vi "Setup.vi"(8 "Error In":errorcluster, 9 "Password":string, 10 "Username":string, 11 "Address":string) -> (0 "Error Out":errorcluster, 3 "Sesssion":refnum<class "Session.lvclass">)   [LabVIEW 2018, in "Tests.lvlib" / "SFTP.lvlib"]
uses:
  SFTP.lvlib
  src/Toolkit/API/Session/Session.lvclass
  src/Toolkit/API/Session/Support/Password Authentication.vi
  src/Toolkit/API/SSH/SSH.lvclass
  Tests.lvlib
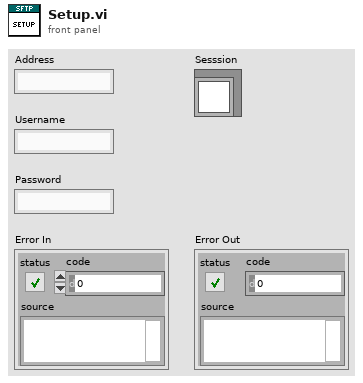
[diagram p1: front panel]
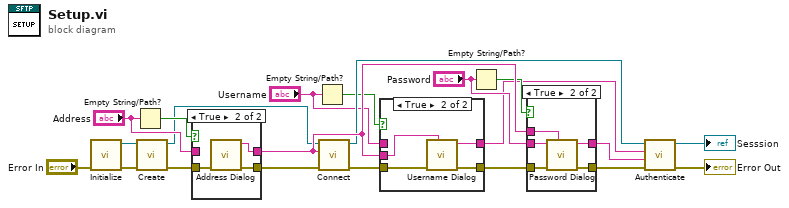
[diagram p0: block diagram]
diagram:
  n1 = call "Initialize.vi"("Error In"="Error In") -> ("Error Out"=w2:errorcluster, "SSH"=w3:refnum<class "SSH.lvclass">)  [unwired: 9 in]
  n2 = Empty String/Path?(string/path="Address") -> (empty?=w6:bool)
  n3 = call "Create.vi"("Error In"=w2, "SSH"=w3) -> ("Error Out"=w8:errorcluster, "Sesssion"=w5:refnum<class "Session.lvclass">)  [unwired: 8 in]
  n4 = case shown="True" w6 {
    tunnel: w8 -> [w22 w26]
    tunnel: [w22 w25] -> w9
    tunnel: [w23 w24] -> w21
    tunnel: "Address" -> [w23 _]
    frame False {
    }
    frame True {
      n5 = call "Address Dialog.vi"("Error In"=w26) -> ("Error Out"=w25:errorcluster, "Address Out"=w24:string)  [unwired: 9 in]
    }
  }
  n6 = Empty String/Path?(string/path="Username") -> (empty?=w15:bool)
  n7 = call "Connect.vi"("Error In"=w9, "Address"=w21, "Session In"=w5) -> ("Error Out"=w18:errorcluster, "Sesssion Out"=w20:refnum<class "Session.lvclass">)  [unwired: 7 in]
  n8 = case shown="True" w15 {
    tunnel: w18 -> [w28 w32]
    tunnel: [w27 w31] -> w13
    tunnel: [w28 w30] -> w10
    tunnel: "Username" -> [w27 _]
    tunnel: w21 -> [_ w29]
    frame False {
    }
    frame True {
      n9 = call "Username Dialog.vi"("Address"=w29, "Error In"=w32) -> ("Error Out"=w30:errorcluster, "Username Out"=w31:string)  [unwired: 8 in]
    }
  }
  n10 = Empty String/Path?(string/path="Password") -> (empty?=w17:bool)
  n11 = case shown="True" w17 {
    tunnel: "Password" -> [w34 w39]
    tunnel: w10 -> [w33 w38]
    tunnel: [w33 w37] -> w11
    tunnel: [w34 w36] -> w12
    tunnel: w21 -> [_ w35]
    frame False {
    }
    frame True {
      n12 = call "Password Dialog.vi"("Address"=w35, "Error In"=w38, "Password In"=w39) -> ("Error Out"=w37:errorcluster, "Password Out"=w36:string)  [unwired: 7 in]
    }
  }
  n13 = call-poly "Authenticate.vi"("Error In"=w11, "Password"=w12, "Username"=w13, "Session In"=w20) -> ("Error Out"=→"Error Out":errorcluster, "Sesssion Out"=→"Sesssion":refnum<class "Session.lvclass">)  [unwired: 6 in]
